vi "back_propagation.vi"(5 "Targets":dbl[][](array[numeric]), 6 "Old Weights":cluster{"Array":dbl[][]}[](array[cluster]), 7 "Neurons":cluster{"Array 2":cluster{"Array":dbl[]}[]}[](array[cluster]), 9 "Input Data":dbl[][](array[numeric]), 10 "# hidden layers":i32, 11 "Learning rate":dbl=0.01 step=0.005) -> (4 "New Weights":cluster{"Array":dbl[][]}[](array[cluster]))   [LabVIEW 2016]
uses:
  <vilib>/Analysis/baseanly.llb/Real Outer Product.vi
  <vilib>/Analysis/baseanly.llb/Vector x A.vi
  <vilib>/Analysis/Matrix/Numeric/Conversions/Matrix To Array - RM.vi
  <vilib>/Analysis/NI_AALBase.lvlib
  <vilib>/Analysis/Matrix/NI_Matrix.lvlib
panel:
  # "Back Propagation unit"
  # "Author: Adam Cavatassi, McGill University, 2018"
  # "Inputs"
  # "Outputs"
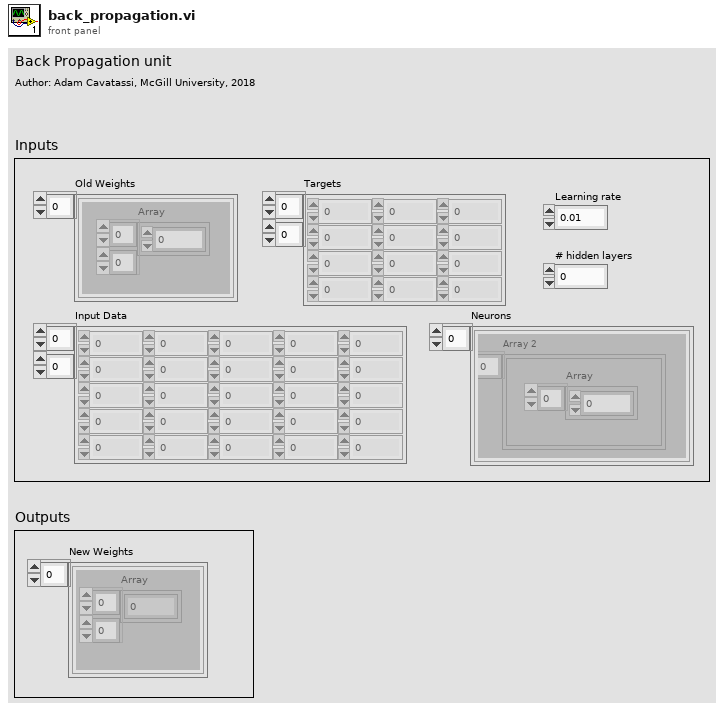
[diagram p1: front panel]
types:
  T1 = typedef "NI_Matrix.lvlib/RealMatrix.ctl" = dbl[][]
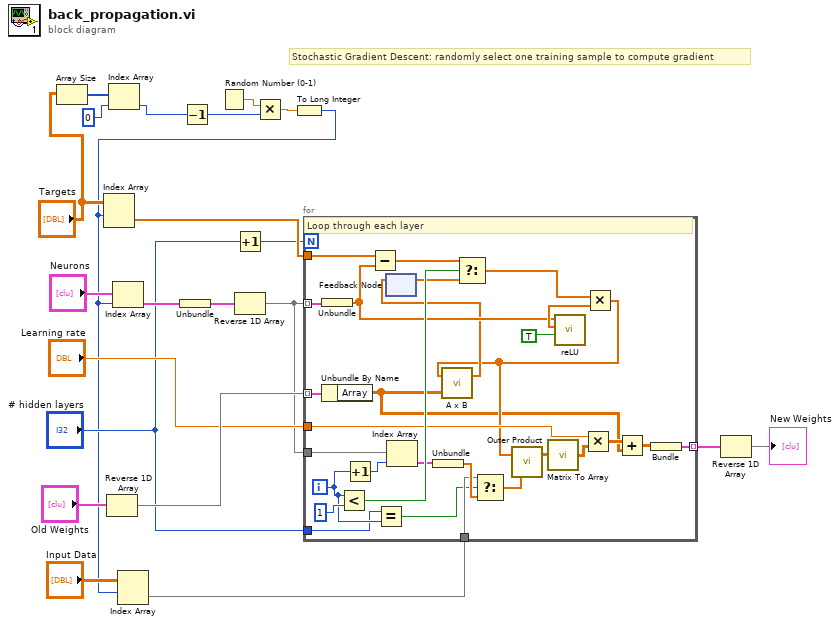
[diagram p0: block diagram]
diagram:
  # "Stochastic Gradient Descent: randomly select one training sample to compute gradient"
  n1 = Array Size(array="Targets") -> (size(s)=w22:i32[])
  n2 = Reverse 1D Array(array="Old Weights") -> (reversed array=w19:cluster{"Array":dbl[][]}[])
  n3 = Index Array(array=w22, index=0) -> (element=w7:i32)
  n4 = Decrement(x=w7) -> (x-1=w1:i32)
  n5 = Random Number (0-1)() -> (number: 0 to 1=w17:dbl)
  n6 = Increment(x="# hidden layers") -> (x+1=w8:i32)
  n7 = Multiply(x=w17, y=w1) -> (x*y=w9:dbl)
  n8 = To Long Integer(number=w9) -> (32bit integer=w2:i32)
  n9 = Index Array(array="Targets", index (row)=w2) -> (element=w10:dbl[])  [unwired: 1 in]
  n10 = Index Array(array="Neurons", index=w2) -> (element=w11:cluster{"Array 2":cluster{"Array":dbl[]}[]})
  n11 = Index Array(array="Input Data", index (row)=w2) -> (element=w6:dbl[])  [unwired: 1 in]
  n12 = Unbundle(w11) -> ("Array 2"=w16:cluster{"Array":dbl[]}[])
  n13 = Reverse 1D Array(array=w16) -> (reversed array=w15:cluster{"Array":dbl[]}[])
  n14 = for {
    N: w8 -> [_]
    tunnel: w10 -> [w51]
    tunnel: w19 -> [w48] mode=indexing
    tunnel: w15 -> [w40] mode=indexing
    tunnel: w15 -> [w39]
    tunnel: "Learning rate" -> [w36]
    tunnel: [w33] -> w4 mode=indexing
    tunnel: w6 -> [w31]
    tunnel: "# hidden layers" -> [w28]
    i -> [w29]
    # "Loop through each layer"
    n15 = Unbundle(w40) -> ("Array"=w43:dbl[])
    n16 = Unbundle By Name(w48) -> ("Array"=w23:dbl[][])
    n17 = Less?(x=w29, y=1) -> (x < y?=w44:bool)
    n18 = Increment(x=w29) -> (x+1=w38:i32)
    n19 = Subtract(x=w51, y=w43) -> (x-y=w47:dbl[])
    n20 = Equal?(x=w28, y=w29) -> (x = y?=w30:bool)
    n21 = feedback #1() -> (w41:dbl[])  [unwired: 1 in]
    n22 = Index Array(array=w39, index=w38) -> (element=w37:cluster{"Array":dbl[]})
    n23 = Unbundle(w37) -> ("Array"=w32:dbl[])
    n24 = Select(t=w47, s=w44, f=w41) -> (s? t:f=w46:dbl[])
    n25 = Select(t=w31, s=w30, f=w32) -> (s? t:f=w27:dbl[])
    n26 = call "reLU.vi"("Derivative?"=TRUE, "Input"=w43) -> ("Output"=w50:dbl[])  [unwired: 9 in]
    n27 = Multiply(x=w46, y=w50) -> (x*y=w26:dbl[])
    n28 = call-poly <vilib>:"A x B.vi"("Matrix A"=w23, "Vector V'"=w26) -> ("V' x A"=w42:dbl[])  [unwired: 1 out]
    n29 = feedback-in #1(w42) -> ()
    n30 = call-poly <vilib>:"Outer Product.vi"("Y Vector"=w27, "X Vector"=w26) -> ("Outer Product"=w25:T1)  [unwired: 1 out]
    n31 = call-poly <vilib>:"Matrix To Array.vi"("Real Matrix"=w25) -> ("Real 2D Array"=w24:dbl[][])
    n32 = Multiply ("Multiply.vi")(x=w36, y=w24) -> (x*y=w35:dbl[][])
    n33 = Add ("Add.vi")(x=w35, y=w23) -> (x+y=w34:dbl[][])
    n34 = Bundle(w34) -> (w33:cluster{dbl[][]})  [unwired: 1 in]
  }
  n35 = Reverse 1D Array(array=w4) -> (reversed array=→"New Weights":cluster{dbl[][]}[])
